vi "niDCPower Get Connections - 1Pin1Connection.vi"(8 "error in":errorcluster, 9 "site":i32=-1, 10 "pin or relay name":string, 11 "session reservation in":refnum<class "Session Reservation.lvclass">) -> (0 "error out":errorcluster, 2 "connection":T1, 3 "session reservation out":refnum<class "Session Reservation.lvclass">)   [LabVIEW 2020, in "MeasurementLink niDCPower.lvlib"]
uses:
  MeasurementLink niDCPower.lvlib
  MeasurementLink Session Management/Session Reservation/Session Reservation.lvclass
  niDCPower Connection.ctl
  MeasurementLink Session Management/Session Reservation/Hardware Independent Connection.ctl
  86b200b6-28cb-4bb1-b3a2-edbec9fb38cc.vi
  86b200b6-28cb-4bb1-b3a2-edbec9fb38cc.vi/d089b476-b30c-4b91-b2ff-fbae0086b065.vi
  MeasurementLink Session Management/Session Reservation/Get Connections Impl.vi
  <vilib>/Utility/error.llb/Error Cluster From Error Code.vi
  Instrument/Instrument.lvclass
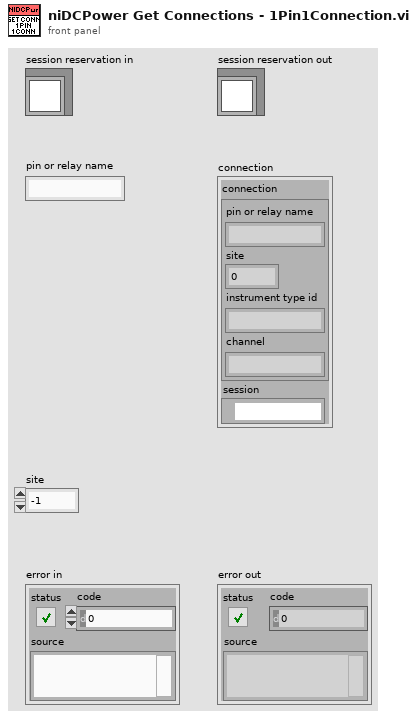
[diagram p1: front panel]
types:
  T1 = typedef "MeasurementLink niDCPower.lvlib/niDCPower Connection.ctl" = cluster{"connection":T2, "session":refnum<k15>}
  T2 = typedef "MeasurementLink Session Management.lvlib/Session Reservation.lvclass/Hardware Independent Connection.ctl" = cluster{"pin or relay name":string, "site":i32, "instrument type id":string, "channel":string}
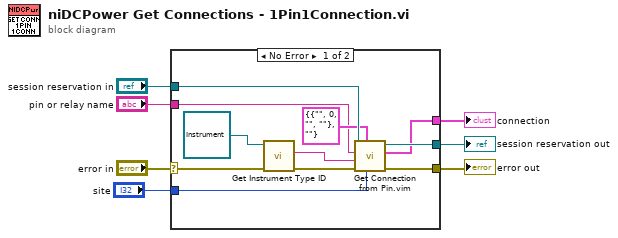
[diagram p0: block diagram]
diagram:
  n1 = case shown="No Error" "error in" {
    selector: "error in" -> [w9 w19]
    tunnel: "session reservation in" -> [w15 w20]
    tunnel: "pin or relay name" -> [w12 _]
    tunnel: [w16 w19] -> w4
    tunnel: [w18 w20] -> w3
    tunnel: [w17 _] -> w2
    tunnel: "site" -> [w14 _]
    frame No Error {
      n2 = call-dynamic "Get Instrument Type ID.vi"("error in"=w9, "instrument in"=refnum<class "Instrument.lvclass"> refnum ("MeasurementLink niDCPower.lvlib:Instrument.lvclass")) -> ("error out"=w8:errorcluster, "instrument type id"=w10:string)  [unwired: 7 in, 1 out]
      n3 = call "Get Connection from Pin.vim"("site"=w14, "connection type"=T1 {"connection"={"pin or relay name"="", "site"=0, "instrument type id"="", "channel"=""}, "session"=""} ("niDCPower connection"), "error in"=w8, "instrument type id"=w10, "pin or relay name"=w12, "session reservation in"=w15) -> ("error out"=w16:errorcluster, "connection"=w17:T1, "session reservation out"=w18:refnum<class "Session Reservation.lvclass">)  [unwired: 3 in]
    }
    frame Error {
    }
  }
  "error out" <- w4
  "session reservation out" <- w3
  "connection" <- w2
